vi "Set Target Attacker.vi"(7 "GOAL":dbl[](array[numeric]), 9 "Position":dbl[](array[numeric]), 11 "Target":dbl[](array[numeric])) -> (1 "output":dbl[](array[numeric]))   [LabVIEW 2016]
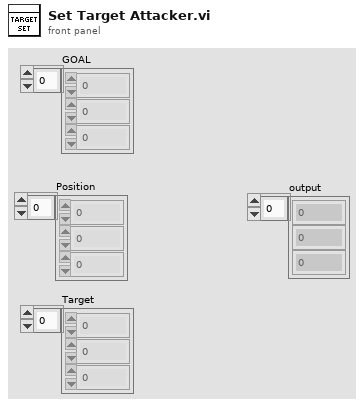
[diagram p1: front panel]
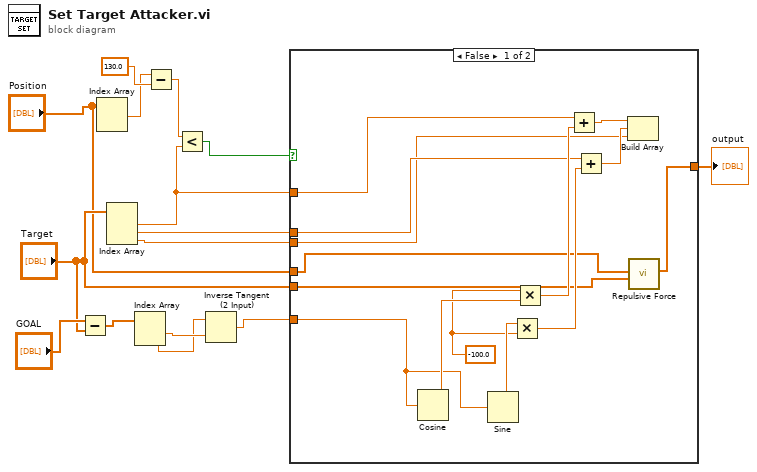
[diagram p0: block diagram]
diagram:
  n1 = Subtract(x="GOAL", y="Target") -> (x-y=w12:dbl[])
  n2 = Index Array(array="Position") -> (element #1=w4:dbl)  [unwired: 2 in, 1 out]
  n3 = Index Array(array="Target") -> (element #1=w8:dbl, element #2=w7:dbl, element #3=w6:dbl)  [unwired: 3 in]
  n4 = Index Array(array=w12) -> (element #1=w11:dbl, element #2=w10:dbl)  [unwired: 2 in]
  n5 = Subtract(x=w4, y=130.0) -> (x-y=w3:dbl)
  n6 = Less?(x=w3, y=w8) -> (x < y?=w15:bool)
  n7 = Inverse Tangent (2 Input)(1:w11, 2:w10) -> (0:w9:dbl)
  n8 = case shown="False" w15 {
    tunnel: [w18 w30] -> w14
    tunnel: w9 -> [w27 _]
    tunnel: w8 -> [w26 _]
    tunnel: w7 -> [w24 _]
    tunnel: w6 -> [w20 _]
    tunnel: "Target" -> [w19 w30]
    tunnel: "Position" -> [w16 _]
    frame False {
      w17 = -100.0 ("y")
      n9 = Cosine(x=w27) -> (cos(x)=w29:dbl)
      n10 = Sine(x=w27) -> (sin(x)=w28:dbl)
      n11 = Multiply(x=w28, y=w17) -> (x*y=w23:dbl)
      n12 = Multiply(x=w17, y=w29) -> (x*y=w25:dbl)
      n13 = Add(x=w26, y=w25) -> (x+y=w22:dbl)
      n14 = Add(x=w24, y=w23) -> (x+y=w21:dbl)
      n15 = Build Array(w22, w21, w20) -> ()  [unwired: 1 out]
      n16 = call "Repulsive Force.vi"("Target"=w19, "Robot Position"=w16) -> ("out"=w18:dbl[])  [unwired: 9 in]
    }
    frame True {
    }
  }
  "output" <- w14
